vi "LSCI 370 Data Heater Output.vi"(0 "VISA session":refnum<visa-resource-name>, 11 "error in (no error)":errorcluster) -> (4 "dup VISA session":refnum<visa-resource-name>, 8 "Heater Output":dbl min=0.0 max=100.0 step=1e-05 format="%^.5e", 15 "error out":errorcluster)   [LabVIEW 2016]
doc: "This VI querys the instrument for the heater output in percent."
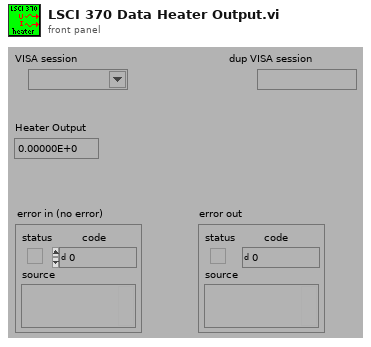
[diagram p1: front panel]
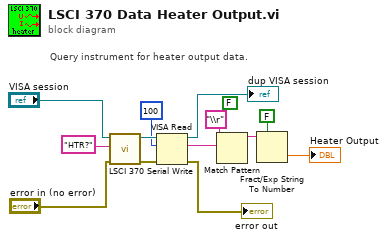
[diagram p0: block diagram]
diagram:
  (unwired) FALSE ("use system decimal point (T)")
  # "Query instrument for heater output data."
  n1 = call "LSCI 370 Serial Write.vi"("error in (no error)"="error in (no error)", "Write Buffer (\"\")"="HTR?", "VISA session"="VISA session") -> ("error out"=w12:errorcluster, "dup VISA session"=w13:refnum<visa-resource-name>)  [unwired: 6 in, 1 out]
  n2 = VISA Read(VISA resource name=w13, byte count=100, error in (no error)=w12) -> (VISA resource name out=→"dup VISA session":refnum<visa-resource-name>, read buffer=w10:string, error out=→"error out":errorcluster)  [unwired: 1 out]
  n3 = Match Pattern(string=w10, regular expression="\\r") -> (before substring=w8:string)  [unwired: 1 in, 3 out]
  n4 = Fract/Exp String To Number(use system decimal point (T)=FALSE, string=w8) -> (number=→"Heater Output":dbl)  [unwired: 2 in, 1 out]
